vi "Display Information.vi"(8 "error in (no error)":errorcluster, 11 "Masterv2 in":refnum<class "Masterv2.lvclass">) -> (0 "error out":errorcluster, 1 "Passwords":string[](array[string]), 3 "Masterv2 out":refnum<class "Masterv2.lvclass">, 4 "Recipe Indicator":string[][](array[string]), 5 "Passwords 2":string[](array[string]))   [LabVIEW 2014, in "Main Libraryv2.lvlib" / "Masterv2.lvclass"]
uses:
  Master/Masterv2.lvclass
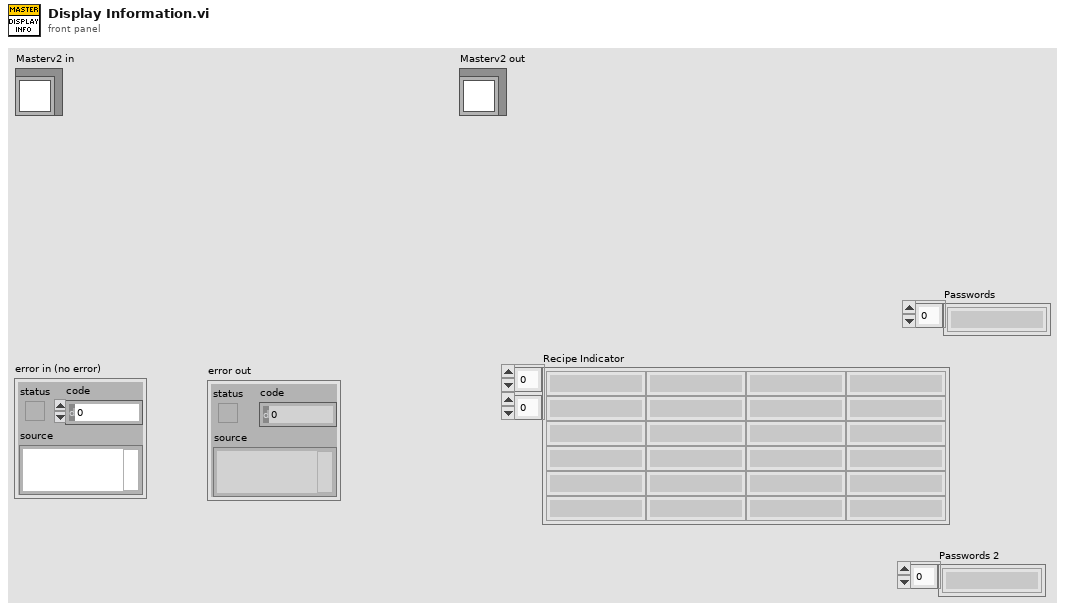
[diagram p1: front panel]
types:
  T1 = cluster{"Speed":string, "Temperature SP":string, "Time Limit":string, "Direction":string}[]
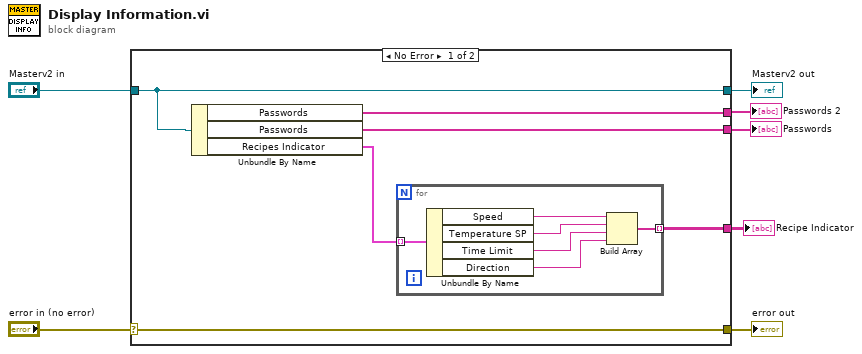
[diagram p0: block diagram]
diagram:
  n1 = case shown="No Error" "error in (no error)" {
    selector: "error in (no error)" -> [w13 w21]
    tunnel: [w13 w21] -> w6
    tunnel: [w9 w20] -> w4
    tunnel: "Masterv2 in" -> [w9 w20]
    tunnel: [w11 _] -> w3
    tunnel: [w10 _] -> w2
    tunnel: [w8 _] -> w1
    frame No Error {
      n2 = Unbundle By Name(w9) -> ("Passwords"=w10:string[], "Passwords"=w8:string[], "Recipes Indicator"=w12:T1)
      n3 = for {
        tunnel: w12 -> [w19] mode=indexing
        tunnel: [w14] -> w11 mode=indexing
        n4 = Unbundle By Name(w19) -> ("Speed"=w18:string, "Temperature SP"=w17:string, "Time Limit"=w16:string, "Direction"=w15:string)
        n5 = Build Array(w18, w17, w16, w15) -> (w14:string[])
      }
    }
    frame Error {
    }
  }
  "error out" <- w6
  "Masterv2 out" <- w4
  "Recipe Indicator" <- w3
  "Passwords" <- w1
  "Passwords 2" <- w2
